vi "Control - Generic - Throttle Closed Loop Host.vi"() -> ()   [LabVIEW 2015, in "ECS-Host.lvlib"]
uses:
  ECS-Host.lvlib
panel:
  in  "AirFlowPID_PIDE":bool
  out "ThrottlePsn_Calc":sgl caption="[mg/cyc]"
  out "AirFlowPID_PIDOut":sgl caption="[mg/cyc]"
  out "ThrottlePsn_FF":sgl caption="[mg/cyc]"
  in  "ThrottleDiameter":sgl caption="[%Open]"
  in  "ThrottleCtrlMode":bool
  in  "ClosedAngle":sgl caption="[%Open]"
  in  "DischargeCoeff":sgl caption="[%Open]"
  in  "AirFlowPID_Td":sgl caption="[]"
  in  "AirFlowPID_Ti":sgl caption="[]"
  in  "AirFlowPID_Kp":sgl caption="[]"
  in  "AirFlowPID_PIDMin":sgl caption="[]"
  in  "AirFlowPID_PIDMax":sgl caption="[mg/cyc]"
  in  "ThrottlePsn_ManE":bool
  in  "ThrottlePsn_Man":sgl caption="[%Open]"
  out "ThrottlePsn_Des":sgl caption="[%Open]"
  # "+"
  # "="
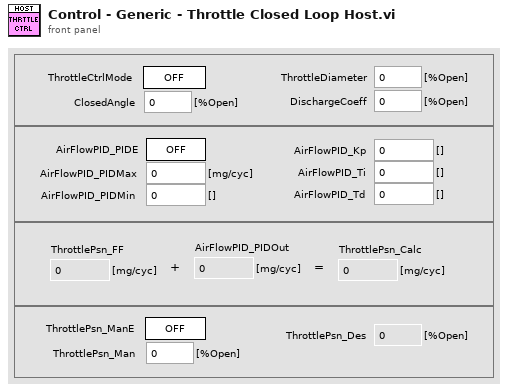
[diagram p1: front panel]
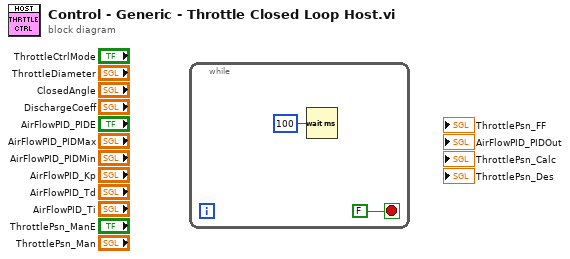
[diagram p0: block diagram]
diagram:
  n1 = while {
    stop <- FALSE stop-if-true
    n2 = Wait (ms)(milliseconds to wait=u32 100) -> ()  [unwired: 1 out]
  }
